vi "DAQ_Cnt_Open.vi"(0 "reference in":refnum<class "DAQ_Base.lvclass">, 5 "error in (no error)":errorcluster) -> (14 "reference out":refnum<class "DAQ_Base.lvclass">, 19 "error out":errorcluster)   [LabVIEW 2020, in "DAQ.lvlib" / "DAQ_Base.lvclass"]
uses:
  DAQ_Base.lvclass
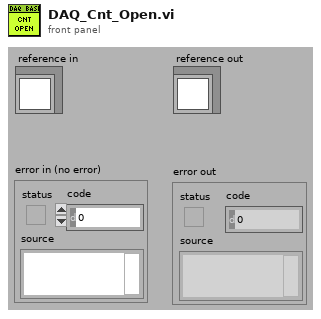
[diagram p1: front panel]
types:
  T1 = typedef "DAQ.lvlib/DAQ_Base.lvclass/ObjectAttributesRef.ctl" = refnum<data-value>
  T2 = typedef "DAQ.lvlib/DAQ_Base.lvclass/ObjectAttributes.ctl" = cluster{"MyAttribute":dbl, "RootPath":path, "DAQSettings":T3, "DaqCollector":cluster{"CollectDataQueue":refnum<queue>, "ArryDataCollectorChannel":T9[], "RealTimeValues":dbl[]}, "CollectorChannelEnable":bool[]}
  T3 = typedef "DAQ.lvlib/DAQ_Base.lvclass/DAQSettings.ctl" = cluster{"SampleSettings":T4, "AI_ChannelSettings":T5, "AO_ChannelSettings":T7, "Cnt_ChannelSettings":T8}
  T4 = typedef "DAQ.lvlib/DAQ_Base.lvclass/SampleSettings.ctl" = cluster{"samples per channel":i32, "SampleRate":dbl, "TansMaxLength":dbl, "ReadTimeOut":dbl, "时钟源":tag}
  T5 = typedef "DAQ.lvlib/DAQ_Base.lvclass/AI_ChannelSettings.ctl" = cluster{"AI_SettingsArry":cluster{"DeviceName":tag, "physical channels":tag, "AssignName":string, "输入信号类型":T6, "Max_value":dbl, "Min_value":dbl, "单位":i32, "shunt resistor location":i32, "external shunt resistor value":dbl, "标定系数":cluster{"Scale":dbl, "Offset":dbl}}[]}
  T6 = typedef "AI信号类型.ctl" = i32
  T7 = typedef "DAQ.lvlib/DAQ_Base.lvclass/AO_ChannelSettings.ctl" = cluster{"布尔":bool}
  T8 = typedef "DAQ.lvlib/DAQ_Base.lvclass/Cnt_ChannelSettings.ctl" = cluster{"Cnt_ChannelSettings":cluster{"类型":enum16{"Linear", "Rotate"}, "CounterNbr":tag, "AssignName":string, "单位":u16, "decoding type":u16, "PPR_DistancePerPulse":dbl, "Initial Position ":dbl, "z index enable":bool, "z index phase":i32, "source":tag}[]}
  T9 = typedef "DAQ.lvlib/DAQ_Base.lvclass/DataCollector.ctl" = cluster{"DataCollectArry":dbl[][], "Update":bool}
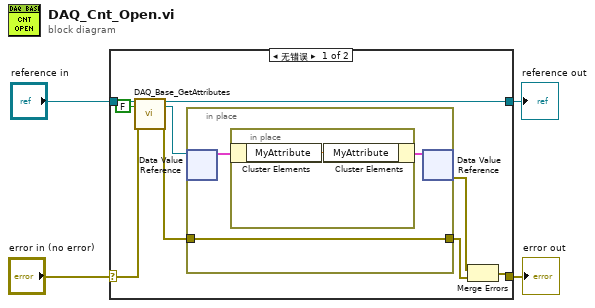
[diagram p0: block diagram]
diagram:
  n1 = case shown="无错误" "error in (no error)" {
    selector: "error in (no error)" -> [w13 w19]
    tunnel: [w5 w19] -> w3
    tunnel: [w12 w18] -> w1
    tunnel: "reference in" -> [w11 w18]
    frame No Error {
      n2 = call "DAQ_Base_GetAttributes.vi"("reference in"=w11, "return data? (T)"=FALSE, "error in (no error)"=w13) -> ("reference out"=w12:refnum<class "DAQ_Base.lvclass">, "attributes ref"=w9:T1, "error out"=w8:errorcluster)  [unwired: 13 in, 1 out]
      n3 = in-place {
        in-place-border: w8 -> [w14]
        in-place-border: [w14] -> w7
        n4 = in-place-dvr #1(w9) -> (w15:T2)  [unwired: 1 out]
        n5 = in-place {
          n6 = in-place-cluster #2(w15) -> ("MyAttribute"=w17:dbl)
          n7 = in-place-cluster #2("MyAttribute"=w17) -> (w16:T2)
        }
        n8 = in-place-dvr #1(w16) -> (w6:errorcluster)  [unwired: 1 out]
      }
      n9 = Merge Errors(w6, w7) -> (w5:errorcluster)
    }
    frame Error {
    }
  }
  "error out" <- w3
  "reference out" <- w1
